vi "Main.vi"(10 "Simulator Bounds":T1={"Simulator E Range"=20.0, "Simulator E Min"=-10.0, "Simulator N Range"=20.0, "Simulator N Min"=-10.0}) -> ()   [LabVIEW 2011]
doc: "The main VI for Sense, Think and Act that controls the sailbot. Also includes logging code and code for communication with the OCU.\nby Olin Sailbot\noriginally by Jason Curtis"
uses:
  2-Think/2 Globals/2 Global.vi
  2-Think/2 Typedefs/eStopCommand.ctl
  <vilib>/Platform/TimedLoop/XDataNode/XDataNode.xnode
  <vilib>/Platform/TimedLoop/XDataNode/nitl_modes.ctl
  <vilib>/Platform/TimedLoop/XDataNode/XDNodeRunTimeDep.lvlib
  <vilib>/Platform/TimedLoop/XDataNode/wakeup.ctl
  <vilib>/Platform/TimedLoop/XDataNode/timing_clust.ctl
  0x2-OCU-Think Comm/0x2 Classes/NetworkStreams/Writer/NetworkStreamWriter.lvclass
  0x2-OCU-Think Comm/0x2 Classes/NetworkStreams/Reader/NetworkStreamReader.lvclass
  0x2-OCU-Think Comm/0x2 Typedefs/ocuCommands.ctl
  0x2-OCU-Think Comm/0x2 Typedefs/ocuMessage.ctl
  2-Think/2 Classes/Logger/Logger.lvclass
  2-Think/2 Globals/2 Message Logger.vi
  2-Think/2 Typedefs/Which Boat.ctl
  2-Think/2 Typedefs/setpoints to boat.ctl
  2-Think/2 Typedefs/rudder angle.ctl
  2-Think/2 Typedefs/sail setpt.ctl
  2-Think/2 Typedefs/UTM Circle.ctl
  2-Think/2 Typedefs/Velocity.ctl
  1,3 B-Simulation/1,3 B Typedefs/simulator bounds.ctl
panel:
  in  "Enable logging?":bool
  in  "Data storage folder":path
  out "Boat Type":T2=enum."Simulation"
  out "E-stop freq.":dbl
  out "Act freq.":dbl
  out "Sense freq.":dbl
  out "Think freq.":dbl
  in  "E-Stop":bool
  # "this is the parent VI under which \nSense Think and Act run."
  # "Will save to U:\\Logs when run on the RIO"
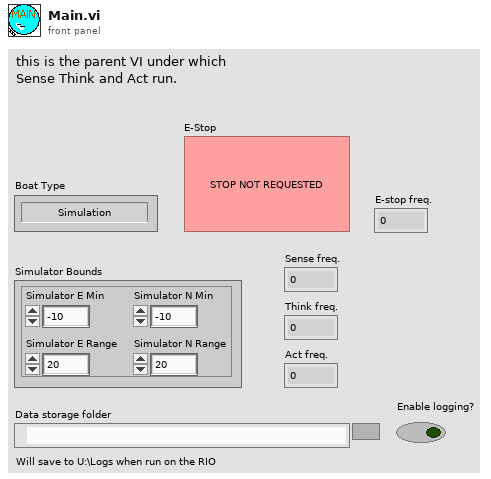
[diagram p1: front panel]
types:
  T1 = typedef "simulator bounds.ctl" = cluster{"Simulator E Range":dbl, "Simulator E Min":dbl, "Simulator N Range":dbl, "Simulator N Min":dbl}
  T2 = typedef "Which Boat.ctl" = enum16{"Axiom; Blackbody Radiation", "Simulation"}
  T3 = typedef "Velocity.ctl" = cluster{"East":dbl, "North":dbl}
  T4 = typedef "setpoints to boat.ctl" = cluster{"Sail Position":T5, "Rudder Angle":T6}
  T5 = typedef "sail setpt.ctl" = dbl
  T6 = typedef "rudder angle.ctl" = dbl
  T7 = typedef "eStopCommand.ctl" = enum16{"Reset E-Stop", "Get E-Stop", "Set E-Stop"}
  T8 = typedef "UTM Circle.ctl" = cluster{"UTM Zone":dbl, "Hemisphere":enum16{"North", "South"}, "East":dbl, "North":dbl, "Radius":dbl}
  T9 = typedef "ocuMessage.ctl" = cluster{"OCU Command":T10, "Data":variant}
  T10 = typedef "ocuCommands.ctl" = enum16{"Pass", "Send override", "Set waypoint number", "Stop", "Add Mission", "Reset Missions/Waypts", "Edit Control Values", "Add Global No-Sail", "Log Message"}
  T11 = typedef "XDNodeRunTimeDep.lvlib/timing_clust.ctl" = cluster{"Expected End [f-1]":u64, "Actual End [f-1]":u64, "Finished Late? [f-1]":bool, "Expected End [i-1]":u64, "Actual End [i-1]":u64, "Finished Late? [i-1]":bool, "Expected Start [i]":u64, "Actual Start [i]":u64, "Expected Start [f]":u64, "Actual Start [f]":u64, "Source Name":string, "Structure Name":string, "Period":i64, "Deadline":i64, "Offset":i64, "Start":i64, "Priority":i32, "Timeout":i32, "Mode":T12, "Wakeup Reason":T13, "Error":errorcluster, "Source Type":string, "Secondary Source Type":string, "Global End Time":u64, "Global Start Time":u64, "Frame Duration":u64, "Iteration Duration":u64, "Assigned CPU":i32, "I/O Scan Engine Mode":u32}
  T12 = typedef "XDNodeRunTimeDep.lvlib/nitl_modes.ctl" = enum32{"No Change", "Process missed periods, maintain original phase", "Discard missed periods, maintain original phase", "Process missed periods, ignore original phase", "Discard missed periods, ignore original phase"}
  T13 = typedef "XDNodeRunTimeDep.lvlib/wakeup.ctl" = enum32{"Normal", "Aborted", "Asynchronous wakeup", "Timing source error", "Timed loop error", "Timeout"}
  T14 = typedef "IMAQ Image.ctl" = refnum<image>
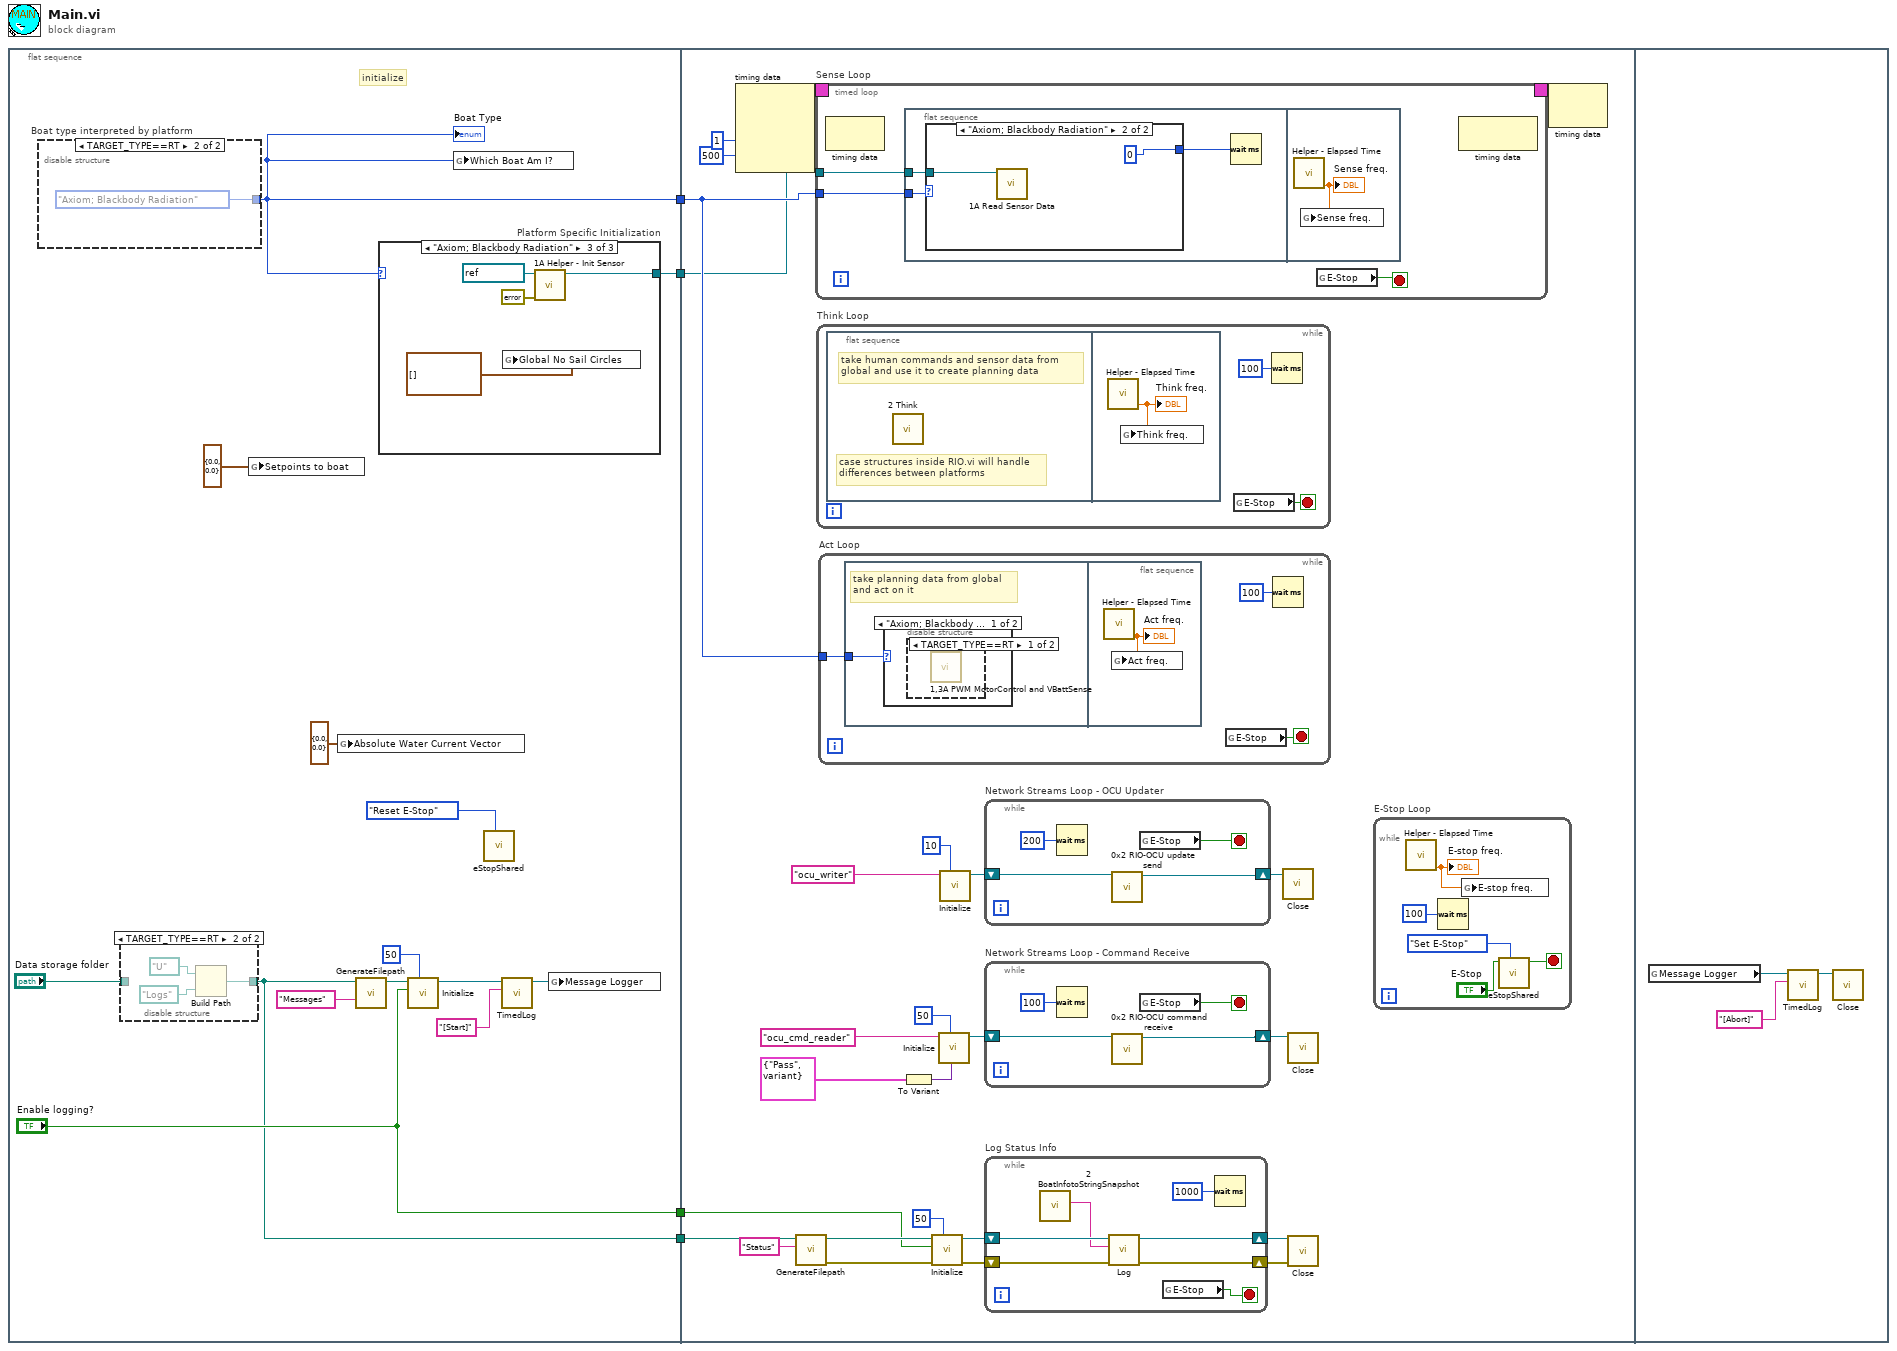
[diagram p0: block diagram]
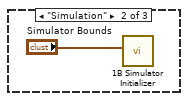
[diagram p3: hidden frame]
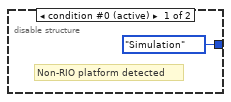
[diagram p5: hidden frame]
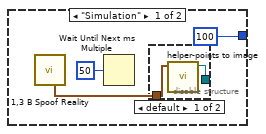
[diagram p6: hidden frame]
diagram:
  n1 = flat-sequence {
    tunnel: [w6] -> w4
    tunnel: [w17] -> w3
    tunnel: [w12] -> w2
    tunnel: ["Enable logging?"] -> w1
    tunnel: w4 -> [w55]
    tunnel: w3 -> [w54]
    tunnel: w2 -> [w38]
    tunnel: w1 -> [w34]
    frame #0 {
      # "initialize"
      n2 = disable-structure "Boat type interpreted by platform" shown="TARGET_TYPE==RT" {
        disable-tunnel: [Which_Boat."Simulation" ("Which Boat Am I?") Which_Boat."Axiom; Blackbody Radiation" ("Which Boat Am I?")] -> w6
        frame condition #0 (active) {
          # "Non-RIO platform detected"
        }
        frame condition #1 {
        }
      }
      "Boat Type" <- w6
      n3 = disable-structure shown="TARGET_TYPE==RT" {
        disable-tunnel: "Data storage folder" -> [w24 _]
        disable-tunnel: [w24 w25] -> w12
        frame condition #0 (active) {
        }
        frame condition #1 {
          n4 = Build Path(base path=path "U:/" ("Data storage folder"), name or relative path=path "Logs" ("Data storage folder")) -> (appended path=w25:path)
        }
      }
      n5 = global write "2 Global.vi" "Setpoints to boat"(T4 {"Sail Position"=0.0, "Rudder Angle"=0.0} ("Setpoints to boat")) -> ()
      n6 = global write "2 Global.vi" "Absolute Water Current Vector"(T3 {"East"=0.0, "North"=0.0} ("Absolute Water Current Vector")) -> ()
      n7 = call "GenerateFilepath.vi"("Identifier"="Messages", "Data storage folder"=w12) -> ("File path out"=w15:path)  [unwired: 8 in, 1 out]
      n8 = case "Platform Specific Initialization" shown="\"Axiom; Blackbody Radiation\"" w6 {
        tunnel: [_ _ w21] -> w17
        frame Default {
        }
        frame "Simulation" {
          n9 = call "1B Simulator Initializer.vi"("Simulator\nBounds"="Simulator Bounds") -> ()  [unwired: 11 in]
        }
        frame "Axiom; Blackbody Radiation" {
          n10 = global write "2 Global.vi" "Global No Sail Circles"(T8[] [] ("Global No Sail Circles")) -> ()
          n11 = call "1A Helper - Init Sensor.vi"("error in (no error)"=errorcluster {"status"=FALSE, "code"=0, "source"=""}, "VISA Refnum in"=refnum<visa-resource-name> "COM1" ("VISA resource name")) -> ("VISA Refnum out"=w21:refnum<visa-resource-name>)  [unwired: 7 in, 2 out]
        }
      }
      n12 = call "Initialize.vi"("buffer size"=50, "Enable? (T)"="Enable logging?", "File path"=w15) -> ("Logger out"=w9:refnum<class "Logger.lvclass">)  [unwired: 7 in, 1 out]
      n13 = global write "2 Global.vi" "Which Boat Am I?"(w6) -> ()
      n14 = call "eStopShared.vi"("Command"=eStopCommand."Reset E-Stop") -> ()  [unwired: 9 in, 2 out]
      n15 = call "TimedLog.vi"("Message"="[Start]", "Logger in"=w9) -> ("Logger out"=w8:refnum<class "Logger.lvclass">)  [unwired: 7 in, 2 out]
      n16 = global write "2 Message Logger.vi" "Message Logger"(w8) -> ()
    }
    frame #1 {
      n17 = node-c288(i64 1 ("Period"), 500 ("Priority")) -> (w33:T11)  [unwired: 2 in]
      n18 = call "GenerateFilepath.vi"("Identifier"="Status", "Data storage folder"=w38) -> ("error out"=w42:errorcluster, "File path out"=w43:path)  [unwired: 8 in]
      n19 = timed-loop "Sense Loop" {
        tunnel: w55 -> [w57]
        tunnel: w54 -> [w56]
        timing: w33 -> [_]
        timing-out: [_] -> w32
        stop <- w58 stop-if-true
        n20 = node-c288() -> ()  [unwired: 1 in, 1 out]
        n21 = flat-sequence {
          tunnel: w56 -> [w61]
          tunnel: w57 -> [w63]
          frame #0 {
            n22 = case shown="\"Axiom; Blackbody Radiation\"" w63 {
              tunnel: [u32 100 ("millisecond multiple") u32 0 ("millisecond multiple")] -> w62
              tunnel: w61 -> [_ w69]
              frame "Simulation" {
                n23 = call "1,3 B Spoof Reality.vi"() -> ("Boat Path"=w65:cluster{"X Position":dbl, "Y Position":dbl}[])  [unwired: 5 in, 6 out]
                n24 = Wait Until Next ms Multiple(millisecond multiple=u32 50) -> ()  [unwired: 1 out]
                n25 = disable-structure shown="default" {
                  disable-tunnel: w65 -> [w68 _]
                  disable-tunnel: [w67 _] -> _
                  frame condition #0 (active) {
                    n26 = call "helper-points to image.vi"("Array of Points"=w68) -> ("Image Out"=w67:T14)  [unwired: 10 in]
                  }
                  frame condition #1 {
                    # "no IMAQ\non RIO"
                  }
                }
              }
              frame "Axiom; Blackbody Radiation" {
                n27 = call "1A Read Sensor Data.vi"("VISA resource name (in)"=w69) -> ()  [unwired: 9 in, 2 out]
              }
            }
            n28 = Wait (ms)(milliseconds to wait=w62) -> ()  [unwired: 1 out]
          }
          frame #1 {
            n29 = call "Helper - Elapsed Time.vi"() -> ("Frequency (Hz)"=w71:dbl)  [unwired: 10 in, 1 out]
            "Sense freq." <- w71
            n30 = global write "2 Global.vi" "Sense freq."(w71) -> ()
          }
        }
        n31 = global read "2 Global.vi" "E-Stop"() -> (w58:bool)
        n32 = node-c288() -> ()  [unwired: 1 in, 1 out]
      }
      n33 = while "Think Loop" {
        stop <- w98 stop-if-true
        n34 = flat-sequence {
          frame #0 {
            # "case structures inside RIO.vi will handle\ndifferences between platforms"
            # "take human commands and sensor data from\nglobal and use it to create planning data"
            n35 = call "2 Think.vi"() -> ()  [unwired: 12 in]
          }
          frame #1 {
            n36 = call "Helper - Elapsed Time.vi"() -> ("Frequency (Hz)"=w99:dbl)  [unwired: 10 in, 1 out]
            "Think freq." <- w99
            n37 = global write "2 Global.vi" "Think freq."(w99) -> ()
          }
        }
        n38 = global read "2 Global.vi" "E-Stop"() -> (w98:bool)
        n39 = Wait (ms)(milliseconds to wait=u32 100 ("millisecond multiple")) -> ()  [unwired: 1 out]
      }
      n40 = while "Act Loop" {
        tunnel: w55 -> [w101]
        stop <- w102 stop-if-true
        n41 = flat-sequence {
          tunnel: w101 -> [w103]
          frame #0 {
            # "take planning data from global\nand act on it"
            n42 = case shown="\"Axiom; Blackbody Radiation\", Default" w103 {
              frame "Axiom; Blackbody Radiation", Default {
                n43 = disable-structure shown="TARGET_TYPE==RT" {
                  frame condition #0 {
                    n44 = call "1,3A PWM MotorControl and VBattSense.vi"() -> ()  [unwired: 12 in]
                  }
                  frame condition #1 (active) {
                  }
                }
              }
              frame "Simulation" {
                # "simulation Act\nis integrated with\nsimulation Think"
              }
            }
          }
          frame #1 {
            n45 = call "Helper - Elapsed Time.vi"() -> ("Frequency (Hz)"=w104:dbl)  [unwired: 10 in, 1 out]
            "Act freq." <- w104
            n46 = global write "2 Global.vi" "Act freq."(w104) -> ()
          }
        }
        n47 = global read "2 Global.vi" "E-Stop"() -> (w102:bool)
        n48 = Wait (ms)(milliseconds to wait=u32 100 ("millisecond multiple")) -> ()  [unwired: 1 out]
      }
      n49 = To Variant(anything=T9 {"OCU Command"=enum."Pass", "Data"=variant} ("OCU Message")) -> (Variant=w49:variant)
      n50 = call "Initialize.vi"("buffer size"=50, "error in (no error)"=w42, "Enable? (T)"=w34, "File path"=w43) -> ("error out"=w39:errorcluster, "Logger out"=w40:refnum<class "Logger.lvclass">)  [unwired: 6 in]
      n51 = call "Initialize.vi"("Default return"=w49, "reader buffer size"=50 ("writer buffer size"), "reader name"="ocu_cmd_reader") -> ("NetworkStreamWriter out"=w45:refnum<class "NetworkStreamReader.lvclass">)  [unwired: 7 in, 1 out]
      n52 = call "Initialize.vi"("writer buffer size"=10, "writer name"="ocu_writer") -> ("NetworkStreamWriter out"=w53:refnum<class "NetworkStreamWriter.lvclass">)  [unwired: 8 in, 1 out]
      n53 = while "Network Streams Loop - OCU Updater" {
        shift-right: [w88] -> w52
        shift-left: w53 -> [w89]
        stop <- w91 stop-if-true
        n54 = Wait (ms)(milliseconds to wait=u32 200 ("millisecond multiple")) -> ()  [unwired: 1 out]
        n55 = call "0x2 RIO-OCU update send.vi"("OCU Writer In"=w89) -> ("OCU Writer Out"=w88:refnum<class "NetworkStreamWriter.lvclass">)  [unwired: 10 in]
        n56 = global read "2 Global.vi" "E-Stop"() -> (w91:bool)
      }
      n57 = while "Network Streams Loop - Command Receive" {
        shift-right: [w84] -> w46
        shift-left: w45 -> [w85]
        stop <- w87 stop-if-true
        n58 = Wait (ms)(milliseconds to wait=u32 100 ("millisecond multiple")) -> ()  [unwired: 1 out]
        n59 = call "0x2 RIO-OCU command receive.vi"("Manual Override Reader In"=w85) -> ("Manual Override Reader Out"=w84:refnum<class "NetworkStreamReader.lvclass">)  [unwired: 10 in]
        n60 = global read "2 Global.vi" "E-Stop"() -> (w87:bool)
      }
      n61 = while "Log Status Info" {
        shift-right: [w81] -> w36
        shift-left: w40 -> [w82]
        shift-right: [w80] -> w35
        shift-left: w39 -> [w79]
        stop <- w83 stop-if-true
        n62 = call "2 BoatInfotoStringSnapshot.vi"() -> ("Snapshot"=w77:string)  [unwired: 11 in]
        n63 = call "Log.vi"("error in (no error)"=w79, "Message"=w77, "Logger in"=w82) -> ("error out"=w80:errorcluster, "Logger out"=w81:refnum<class "Logger.lvclass">)  [unwired: 7 in]
        n64 = global read "2 Global.vi" "E-Stop"() -> (w83:bool)
        n65 = Wait (ms)(milliseconds to wait=u32 1000 ("millisecond multiple")) -> ()  [unwired: 1 out]
      }
      n66 = call "Close.vi"("NetworkStreamWriter in"=w52) -> ()  [unwired: 10 in, 1 out]
      n67 = call "Close.vi"("NetworkStreamReader in"=w46) -> ()  [unwired: 10 in, 1 out]
      n68 = call "Close.vi"("error in (no error)"=w35, "Logger in"=w36) -> ()  [unwired: 9 in, 1 out]
      n69 = while "E-Stop Loop" {
        stop <- w93 stop-if-true
        n70 = call "Helper - Elapsed Time.vi"() -> ("Frequency (Hz)"=w92:dbl)  [unwired: 10 in, 1 out]
        "E-stop freq." <- w92
        n71 = Wait (ms)(milliseconds to wait=u32 100 ("millisecond multiple")) -> ()  [unwired: 1 out]
        n72 = global write "2 Global.vi" "E-stop freq."(w92) -> ()
        n73 = call "eStopShared.vi"("Command"=eStopCommand."Set E-Stop", "E-Stop"="E-Stop") -> ("E-Stop Out"=w93:bool)  [unwired: 8 in, 1 out]
      }
      n74 = node-c288(w32) -> ()  [unwired: 1 out]
    }
    frame #2 {
      n75 = global read "2 Message Logger.vi" "Message Logger"() -> (w107:refnum<class "Logger.lvclass">)
      n76 = call "TimedLog.vi"("Message"="[Abort]", "Logger in"=w107) -> ("Logger out"=w105:refnum<class "Logger.lvclass">)  [unwired: 7 in, 2 out]
      n77 = call "Close.vi"("Logger in"=w105) -> ()  [unwired: 10 in, 1 out]
    }
  }
